vi "proc_demo.vi"() -> ()   [LabVIEW 2011]
panel:
  out "exited":bool
  out "bytes read":i32
  out "bytes to read":i32
  out "string":string
  out "error out":errorcluster
  in  "command":string
  in  "folder":string
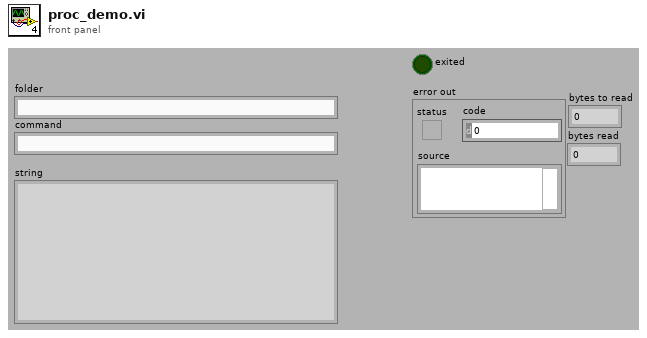
[diagram p1: front panel]
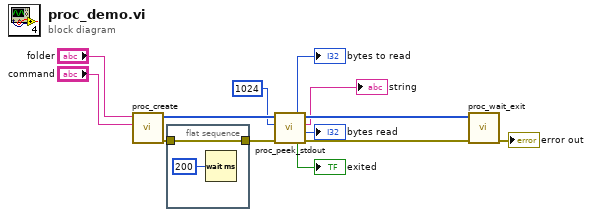
[diagram p0: block diagram]
diagram:
  n1 = call "proc_create.vi"("command"="command", "folder"="folder") -> ("error out"=w2:errorcluster, "process instance handle"=w9:u32[])  [unwired: 8 in]
  n2 = flat-sequence {
    tunnel: [w15] -> w1
    tunnel: w2 -> [w15]
    frame #0 {
      n3 = Wait (ms)(milliseconds to wait=u32 200) -> ()  [unwired: 1 out]
    }
  }
  n4 = call "proc_peek_stdout.vi"("error in"=w1, "size"=1024, "process instance handle in"=w9) -> ("error out"=w11:errorcluster, "bytes read"=→"bytes read":i32, "read buffer"=→"string":string, "process instance handle out"=w10:u32[], "exited"=→"exited":bool, "bytes to read"=→"bytes to read":i32)  [unwired: 3 in]
  n5 = call "proc_wait_exit.vi"("error in"=w11, "process instance handle in"=w10) -> ("error out"=→"error out":errorcluster)  [unwired: 7 in, 2 out]
